vi "Test Parse Temperature from String.vi"(11 "Test Case In":refnum<class "String Parser Test.lvclass">) -> (0 "error out":errorcluster, 3 "Test Case Out":refnum<class "String Parser Test.lvclass">)   [LabVIEW 2020, in "String Parser Test.lvclass"]
uses:
  String Parser Test.lvclass
  C:/Program Files (x86)/National Instruments/LabVIEW 2020/vi.lib/Astemes/LUnit/Test Case.lvclass
  String Parser Test.lvclass/String Parser Test.ctl
  <vilib>/Astemes/LUnit/Test Case.lvclass/Test Case.ctl
  4993e8ee-a06a-463a-9684-69129f64d5ce.vi
  <vilib>/Astemes/LUnit/Append Pass Result.vi
  <vilib>/Astemes/LUnit/Append Fail Result.vi
  <vilib>/Astemes/LUnit/Describe Comparison.vi
  <vilib>/Astemes/LUnit/Compare Variants.vi
  <vilib>/Astemes/LUnit/Run In UI.vi
  <vilib>/Utility/error.llb/Clear Errors.vi
  <vilib>/Astemes/LUnit/Describe Variant.vi
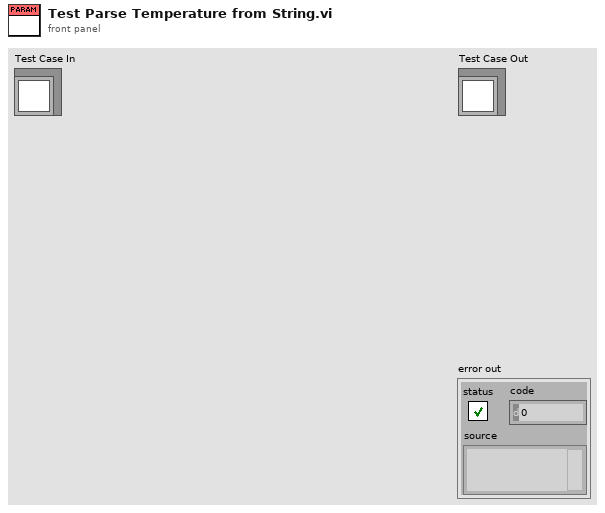
[diagram p1: front panel]
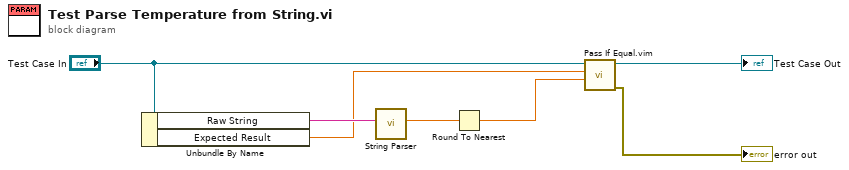
[diagram p0: block diagram]
diagram:
  n1 = Unbundle By Name("Test Case In") -> ("Raw String"=w4:string, "Expected Result"=w2:dbl)
  n2 = call "String Parser.vi"("Raw String"=w4) -> ("Value"=w3:dbl)  [unwired: 10 in]
  n3 = Round To Nearest(number=w3) -> (nearest integer value=w1:dbl)
  n4 = call "Pass If Equal.vim"("Actual"=w1, "Expected"=w2, "LUnit Test Case In"="Test Case In") -> ("error out"=→"error out":errorcluster, "LUnit Test Case Out"=→"Test Case Out":refnum<class "String Parser Test.lvclass">)  [unwired: 7 in]
